vi "BeijingMetro.vi"(9 "终点站":string, 10 "起点站":string) -> (2 "最短站数":i32)   [LabVIEW 2020]
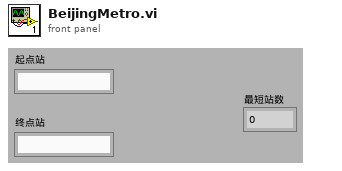
[diagram p1: front panel]
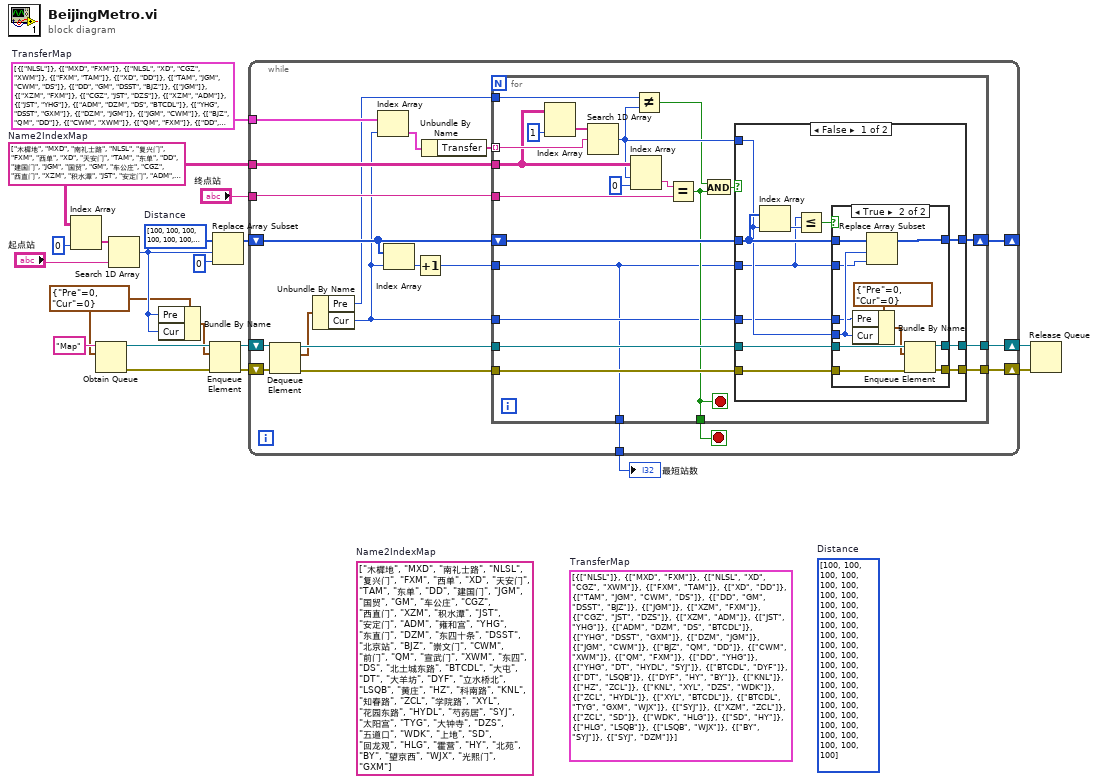
[diagram p0: block diagram]
diagram:
  (unwired) i32[] [100, 100, 100, 100, 100, 100, 100, 100, 100, 100, 100, 100, 100, 100, 100, 100, 100, 100, 100, 100, 100, 100, 100, 100, 100, 100, 100, 100, 100, 100, 100, 100, 100, 100, 100, 100, 100, 100, 100]  # Distance
  (unwired) string[][] [["木樨地", "MXD"], ["南礼士路", "NLSL"], ["复兴门", "FXM"], ["西单", "XD"], ["天安门", "TAM"], ["东单", "DD"], ["建国门", "JGM"], ["国贸", "GM"], ["车公庄", "CGZ"], ["西直门", "XZM"], ["积水潭", "JST"], ["安定门", "ADM"], ["雍和宫", "YHG"], ["东直门", "DZM"], ["东四十条", "DSST"], ["北京站", "BJZ"], ["崇文门", "CWM"], ["前门", "QM"], ["宣武门", "XWM"], ["东四", "DS"], ["北土城东路", "BTCDL"], ["大屯", "DT"], ["大羊坊", "DYF"], ["立水桥北", "LSQB"], ["黄庄", "HZ"], ["科南路", "KNL"], ["知春路", "ZCL"], ["学院路", "XYL"], ["花园东路", "HYDL"], ["芍药居", "SYJ"], ["太阳宫", "TYG"], ["大钟寺", "DZS"], ["五道口", "WDK"], ["上地", "SD"], ["回龙观", "HLG"], ["霍营", "HY"], ["北苑", "BY"], ["望京西", "WJX"], ["光熙门", "GXM"]]  # Name2IndexMap
  (unwired) cluster{"Transfer":string[]}[] [{"Transfer"=["NLSL"]}, {"Transfer"=["MXD", "FXM"]}, {"Transfer"=["NLSL", "XD", "CGZ", "XWM"]}, {"Transfer"=["FXM", "TAM"]}, {"Transfer"=["XD", "DD"]}, {"Transfer"=["TAM", "JGM", "CWM", "DS"]}, {"Transfer"=["DD", "GM", "DSST", "BJZ"]}, {"Transfer"=["JGM"]}, {"Transfer"=["XZM", "FXM"]}, {"Transfer"=["CGZ", "JST", "DZS"]}, {"Transfer"=["XZM", "ADM"]}, {"Transfer"=["JST", "YHG"]}, {"Transfer"=["ADM", "DZM", "DS", "BTCDL"]}, {"Transfer"=["YHG", "DSST", "GXM"]}, {"Transfer"=["DZM", "JGM"]}, {"Transfer"=["JGM", "CWM"]}, {"Transfer"=["BJZ", "QM", "DD"]}, {"Transfer"=["CWM", "XWM"]}, {"Transfer"=["QM", "FXM"]}, {"Transfer"=["DD", "YHG"]}, {"Transfer"=["YHG", "DT", "HYDL", "SYJ"]}, {"Transfer"=["BTCDL", "DYF"]}, {"Transfer"=["DT", "LSQB"]}, {"Transfer"=["DYF", "HY", "BY"]}, {"Transfer"=["KNL"]}, {"Transfer"=["HZ", "ZCL"]}, {"Transfer"=["KNL", "XYL", "DZS", "WDK"]}, {"Transfer"=["ZCL", "HYDL"]}, {"Transfer"=["XYL", "BTCDL"]}, {"Transfer"=["BTCDL", "TYG", "GXM", "WJX"]}, {"Transfer"=["SYJ"]}, {"Transfer"=["XZM", "ZCL"]}, {"Transfer"=["ZCL", "SD"]}, {"Transfer"=["WDK", "HLG"]}, {"Transfer"=["SD", "HY"]}, {"Transfer"=["HLG", "LSQB"]}, {"Transfer"=["LSQB", "WJX"]}, {"Transfer"=["BY", "SYJ"]}, {"Transfer"=["SYJ", "DZM"]}]  # TransferMap
  w3 = cluster{"Pre":i32, "Cur":i32} {"Pre"=0, "Cur"=0}
  w17 = i32[] [100, 100, 100, 100, 100, 100, 100, 100, 100, 100, 100, 100, 100, 100, 100, 100, 100, 100, 100, 100, 100, 100, 100, 100, 100, 100, 100, 100, 100, 100, 100, 100, 100, 100, 100, 100, 100, 100, 100]  # Distance
  w9 = cluster{"Transfer":string[]}[] [{"Transfer"=["NLSL"]}, {"Transfer"=["MXD", "FXM"]}, {"Transfer"=["NLSL", "XD", "CGZ", "XWM"]}, {"Transfer"=["FXM", "TAM"]}, {"Transfer"=["XD", "DD"]}, {"Transfer"=["TAM", "JGM", "CWM", "DS"]}, {"Transfer"=["DD", "GM", "DSST", "BJZ"]}, {"Transfer"=["JGM"]}, {"Transfer"=["XZM", "FXM"]}, {"Transfer"=["CGZ", "JST", "DZS"]}, {"Transfer"=["XZM", "ADM"]}, {"Transfer"=["JST", "YHG"]}, {"Transfer"=["ADM", "DZM", "DS", "BTCDL"]}, {"Transfer"=["YHG", "DSST", "GXM"]}, {"Transfer"=["DZM", "JGM"]}, {"Transfer"=["JGM", "CWM"]}, {"Transfer"=["BJZ", "QM", "DD"]}, {"Transfer"=["CWM", "XWM"]}, {"Transfer"=["QM", "FXM"]}, {"Transfer"=["DD", "YHG"]}, {"Transfer"=["YHG", "DT", "HYDL", "SYJ"]}, {"Transfer"=["BTCDL", "DYF"]}, {"Transfer"=["DT", "LSQB"]}, {"Transfer"=["DYF", "HY", "BY"]}, {"Transfer"=["KNL"]}, {"Transfer"=["HZ", "ZCL"]}, {"Transfer"=["KNL", "XYL", "DZS", "WDK"]}, {"Transfer"=["ZCL", "HYDL"]}, {"Transfer"=["XYL", "BTCDL"]}, {"Transfer"=["BTCDL", "TYG", "GXM", "WJX"]}, {"Transfer"=["SYJ"]}, {"Transfer"=["XZM", "ZCL"]}, {"Transfer"=["ZCL", "SD"]}, {"Transfer"=["WDK", "HLG"]}, {"Transfer"=["SD", "HY"]}, {"Transfer"=["HLG", "LSQB"]}, {"Transfer"=["LSQB", "WJX"]}, {"Transfer"=["BY", "SYJ"]}, {"Transfer"=["SYJ", "DZM"]}]  # TransferMap
  w8 = string[][] [["木樨地", "MXD"], ["南礼士路", "NLSL"], ["复兴门", "FXM"], ["西单", "XD"], ["天安门", "TAM"], ["东单", "DD"], ["建国门", "JGM"], ["国贸", "GM"], ["车公庄", "CGZ"], ["西直门", "XZM"], ["积水潭", "JST"], ["安定门", "ADM"], ["雍和宫", "YHG"], ["东直门", "DZM"], ["东四十条", "DSST"], ["北京站", "BJZ"], ["崇文门", "CWM"], ["前门", "QM"], ["宣武门", "XWM"], ["东四", "DS"], ["北土城东路", "BTCDL"], ["大屯", "DT"], ["大羊坊", "DYF"], ["立水桥北", "LSQB"], ["黄庄", "HZ"], ["科南路", "KNL"], ["知春路", "ZCL"], ["学院路", "XYL"], ["花园东路", "HYDL"], ["芍药居", "SYJ"], ["太阳宫", "TYG"], ["大钟寺", "DZS"], ["五道口", "WDK"], ["上地", "SD"], ["回龙观", "HLG"], ["霍营", "HY"], ["北苑", "BY"], ["望京西", "WJX"], ["光熙门", "GXM"]]  # Name2IndexMap
  n1 = Index Array(array=w8, index (col)=0 ("disabled index (col)")) -> (element=w19:string[])  [unwired: 1 in]
  n2 = Obtain Queue(name (unnamed)="Map", element data type=w3) -> (queue out=w13:refnum<queue>, error out=w12:errorcluster)  [unwired: 3 in, 1 out]
  n3 = Search 1D Array(1D array=w19, element="起点站") -> (index of element=w4:i32)  [unwired: 1 in]
  n4 = Bundle By Name(cluster=w3, "Pre"=w4, "Cur"=w4) -> (w2:cluster{"Pre":i32, "Cur":i32})
  n5 = Enqueue Element(queue=w13, element=w2, error in (no error)=w12) -> (queue out=w11:refnum<queue>, error out=w10:errorcluster)  [unwired: 1 in, 1 out]
  n6 = Replace Array Subset(array=w17, new element=0 ("new element/subarray"), index=w4) -> (w15:i32[])
  n7 = while {
    shift-right: [w32] -> _
    shift-left: w15 -> [w33]
    tunnel: w9 -> [w38]
    tunnel: w8 -> [w35]
    tunnel: "终点站" -> [w34]
    shift-right: [w28] -> w6
    shift-left: w10 -> [w39]
    shift-right: [w29] -> w5
    shift-left: w11 -> [w40]
    tunnel: [w21] -> w1
    stop <- w27 stop-if-true
    n8 = Dequeue Element(queue=w40, error in (no error)=w39) -> (queue out=w31:refnum<queue>, element=w26:cluster{"Pre":i32, "Cur":i32}, error out=w30:errorcluster)  [unwired: 1 in, 1 out]
    n9 = Unbundle By Name(w26) -> ("Pre"=w25:i32, "Cur"=w24:i32)
    n10 = Index Array(array=w38, index=w24) -> (element=w37:cluster{"Transfer":string[]})
    n11 = Index Array(array=w33, index=w24) -> (element=w23:i32)
    n12 = Increment(x=w23) -> (x+1=w22:i32)
    n13 = Unbundle By Name(w37) -> ("Transfer"=w36:string[])
    n14 = for {
      tunnel: w36 -> [w58] mode=indexing
      tunnel: w35 -> [w56]
      tunnel: w34 -> [w54]
      tunnel: w22 -> [w41]
      tunnel: w31 -> [w52]
      tunnel: w30 -> [w51]
      tunnel: [w50] -> w29
      tunnel: [w49] -> w28
      tunnel: [w44] -> w27
      shift-right: [w53] -> w32
      shift-left: w33 -> [w48]
      tunnel: w25 -> [w47]
      tunnel: w24 -> [w42]
      tunnel: [w41] -> w21
      stop <- w44 stop-if-true
      n15 = Index Array(array=w56, index (col)=1 ("disabled index (col)")) -> (element=w59:string[])  [unwired: 1 in]
      n16 = Search 1D Array(1D array=w59, element=w58) -> (index of element=w46:i32)  [unwired: 1 in]
      n17 = Index Array(array=w56, index (row)=w46, index (col)=0 ("disabled index (col)")) -> (element=w55:string)
      n18 = Not Equal?(x=w47, y=w46) -> (x != y?=w45:bool)
      n19 = Equal?(x=w55, y=w54) -> (x = y?=w44:bool)
      n20 = And(x=w45, y=w44) -> (x .and. y?=w43:bool)
      n21 = case shown="False" w43 {
        tunnel: w48 -> [w66 w88]
        tunnel: w46 -> [w64 _]
        tunnel: [w71 w88] -> w53
        tunnel: w52 -> [w70 w87]
        tunnel: w51 -> [w69 w86]
        tunnel: [w68 w87] -> w50
        tunnel: [w67 w86] -> w49
        tunnel: w42 -> [w63 _]
        tunnel: w41 -> [w61 _]
        frame False {
          n22 = Index Array(array=w66, index=w64) -> (element=w65:i32)
          n23 = Less Or Equal?(x=w61, y=w65) -> (x <= y?=w62:bool)
          n24 = case shown="True" w62 {
            tunnel: [w74 w85] -> w71
            tunnel: w70 -> [w73 w84]
            tunnel: w69 -> [w72 w83]
            tunnel: [w73 w82] -> w68
            tunnel: [w72 w81] -> w67
            tunnel: w66 -> [w74 w80]
            tunnel: w64 -> [_ w79]
            tunnel: w63 -> [_ w78]
            tunnel: w61 -> [_ w75]
            frame False {
            }
            frame True {
              n25 = Bundle By Name(cluster=cluster{"Pre":i32, "Cur":i32} {"Pre"=0, "Cur"=0}, "Pre"=w78, "Cur"=w79) -> (w76:cluster{"Pre":i32, "Cur":i32})
              n26 = Replace Array Subset(array=w80, new element=w75, index=w79) -> (w85:i32[])
              n27 = Enqueue Element(queue=w84, element=w76, error in (no error)=w83) -> (queue out=w82:refnum<queue>, error out=w81:errorcluster)  [unwired: 1 in, 1 out]
            }
          }
        }
        frame True {
        }
      }
    }
  }
  "最短站数" <- w1
  n28 = Release Queue(queue=w5, error in (no error)=w6) -> ()  [unwired: 1 in, 3 out]
